vi "InsertIntoArray.vi"(0 "ROSCO Params":T3, 1 "ArrayPairs":T1={"iStatus"={"Index"=0, "Value"=0.0}, "TIME"={"Index"=1, "Value"=0.0}, "DT"={"Index"=2, "Value"=0.0}, "BL_PITCH"={"Index"=3, "Value"=0.0}, "VS_MECHGENPWR"={"Index"=13, "Value"=0.0}, "VS_GENPWR"={"Index"=14, "Value"=0.0}, "GEN_SPEED"={"Index"=19, "Value"=0.0}, "ROTOR_SPEED"={"Index"=20, "Value"=0.0}, "GENTQMEAS"={"Index"=22, "Value"=0.0}, "Y_M"={"Index"=23, "Value"=0.0}, "HORWINDV"={"Index"=26, "Value"=0.0}, "ROOTMOOP1"={"Index"=29, "Value"=0.0}, "ROOTMOOP2"={"Index"=30, "Value"=0.0}, "BL_PITCH2"={"Index"=32, "Value"=0.0}, "BL_PITCH3"={"Index"=33, "Value"=0.0}, "ROOTMOOP3"={"Index"=31, "Value"=0.0}, "AVCMSG_SIZE"={"Index"=48, "Value"=0.0}, "INFILE_SIZE "={"Index"=49, "Value"=0.0}, "OUTFILE_SIZE "={"Index"=50, "Value"=0.0}, "FA_ACC"={"Index"=52, "Value"=0.0}, "NUM_BLADES"={"Index"=60, "Value"=0.0}, "OUT_BL_PITCH"={"Index"=44, "Value"=0.0}, "OUT_TORQUE"={"Index"=46, "Value"=0.0}, "OUT_AERODYN_TQ"={"Index"=89, "Value"=0.0}}, 3 "error in (no error)":errorcluster, 4 "index":i32, 6 "number":sgl) -> (7 "ROSCO Params Out":T3, 8 "ArrayPairs Out":T1={"iStatus"={"Index"=0, "Value"=0.0}, "TIME"={"Index"=1, "Value"=0.0}, "DT"={"Index"=2, "Value"=0.0}, "BL_PITCH"={"Index"=3, "Value"=0.0}, "VS_MECHGENPWR"={"Index"=13, "Value"=0.0}, "VS_GENPWR"={"Index"=14, "Value"=0.0}, "GEN_SPEED"={"Index"=19, "Value"=0.0}, "ROTOR_SPEED"={"Index"=20, "Value"=0.0}, "GENTQMEAS"={"Index"=22, "Value"=0.0}, "Y_M"={"Index"=23, "Value"=0.0}, "HORWINDV"={"Index"=26, "Value"=0.0}, "ROOTMOOP1"={"Index"=29, "Value"=0.0}, "ROOTMOOP2"={"Index"=30, "Value"=0.0}, "BL_PITCH2"={"Index"=32, "Value"=0.0}, "BL_PITCH3"={"Index"=33, "Value"=0.0}, "ROOTMOOP3"={"Index"=31, "Value"=0.0}, "AVCMSG_SIZE"={"Index"=48, "Value"=0.0}, "INFILE_SIZE "={"Index"=49, "Value"=0.0}, "OUTFILE_SIZE "={"Index"=50, "Value"=0.0}, "FA_ACC"={"Index"=52, "Value"=0.0}, "NUM_BLADES"={"Index"=60, "Value"=0.0}, "OUT_BL_PITCH"={"Index"=44, "Value"=0.0}, "OUT_TORQUE"={"Index"=46, "Value"=0.0}, "OUT_AERODYN_TQ"={"Index"=89, "Value"=0.0}}, 10 "error out":errorcluster)   [LabVIEW 2018]
uses:
  Clusters/RoscoParams.ctl
  Clusters/ArrayPairs.ctl
  Clusters/SwapArrayCluster.ctl
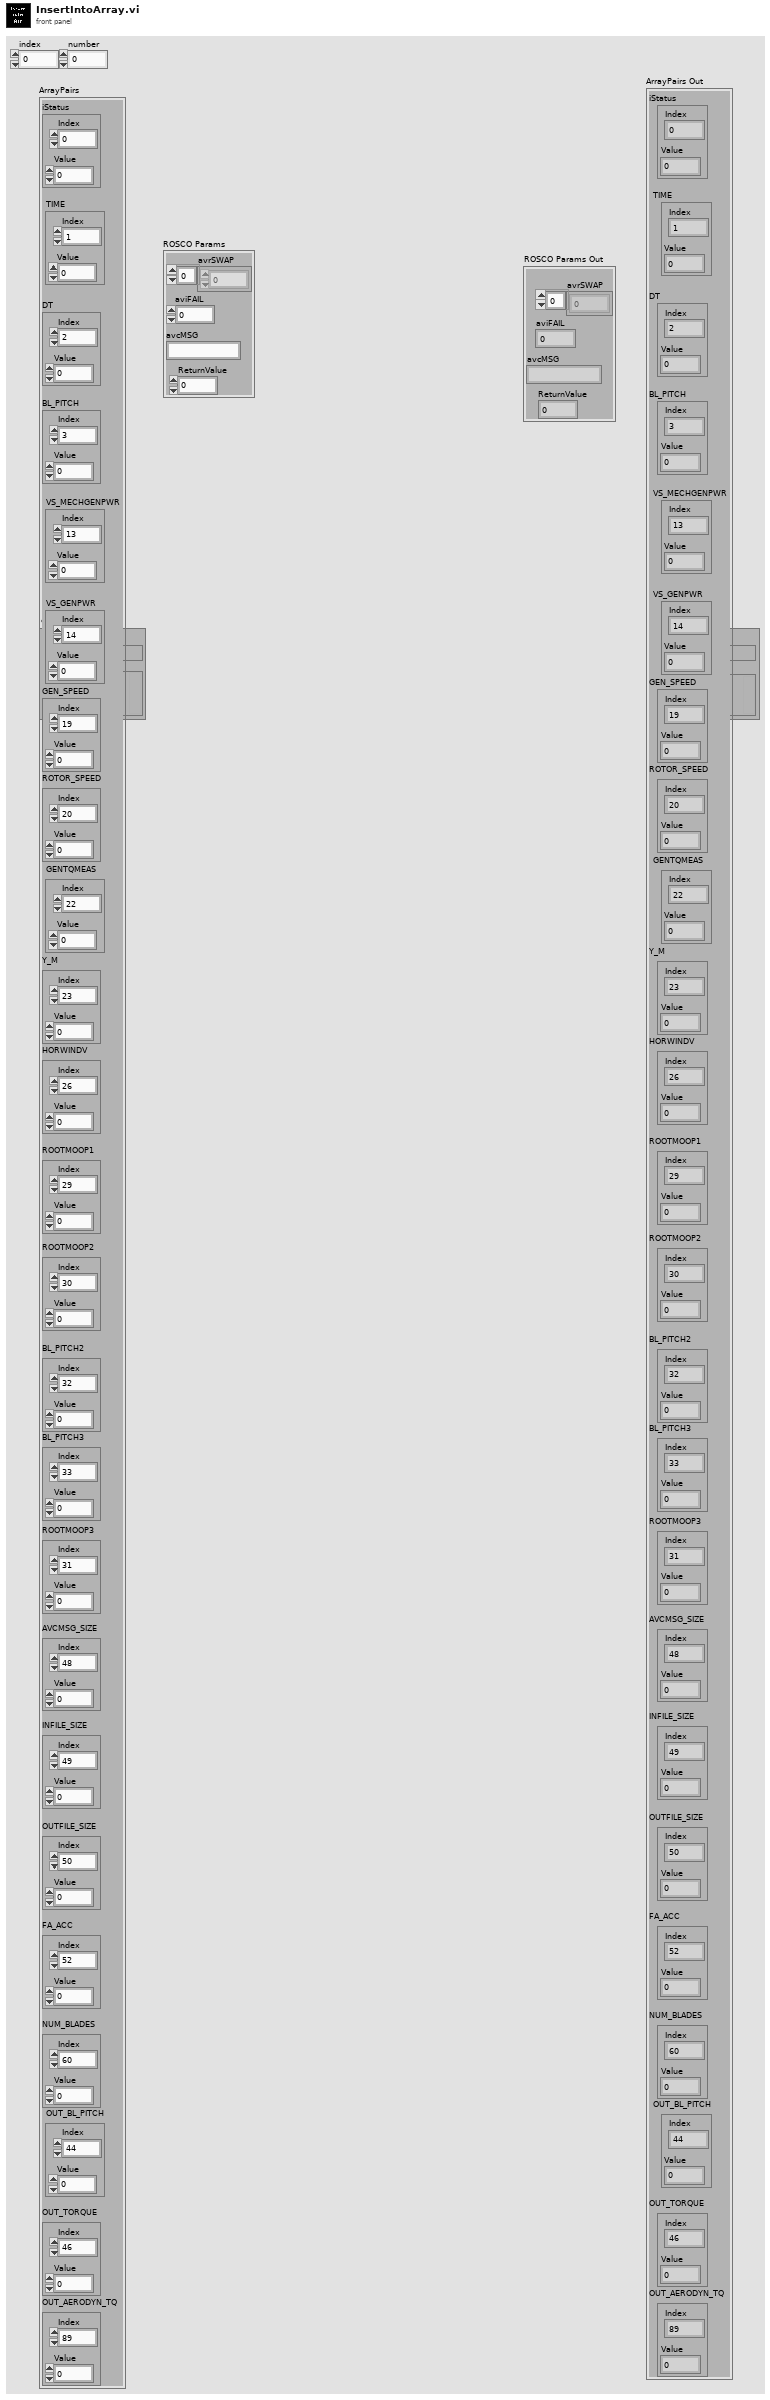
[diagram p1: front panel]
types:
  T1 = typedef "ArrayPairs.ctl" = cluster{"iStatus":T2, "TIME":T2, "DT":T2, "BL_PITCH":T2, "VS_MECHGENPWR":T2, "VS_GENPWR":T2, "GEN_SPEED":T2, "ROTOR_SPEED":T2, "GENTQMEAS":T2, "Y_M":T2, "HORWINDV":T2, "ROOTMOOP1":T2, "ROOTMOOP2":T2, "BL_PITCH2":T2, "BL_PITCH3":T2, "ROOTMOOP3":T2, "AVCMSG_SIZE":T2, "INFILE_SIZE ":T2, "OUTFILE_SIZE ":T2, "FA_ACC":T2, "NUM_BLADES":T2, "OUT_BL_PITCH":T2, "OUT_TORQUE":T2, "OUT_AERODYN_TQ":T2}
  T2 = typedef "SwapArrayCluster.ctl" = cluster{"Index":i32, "Value":sgl}
  T3 = typedef "RoscoParams.ctl" = cluster{"avrSWAP":sgl[], "aviFAIL":i32, "avcMSG":string, "ReturnValue":i32}
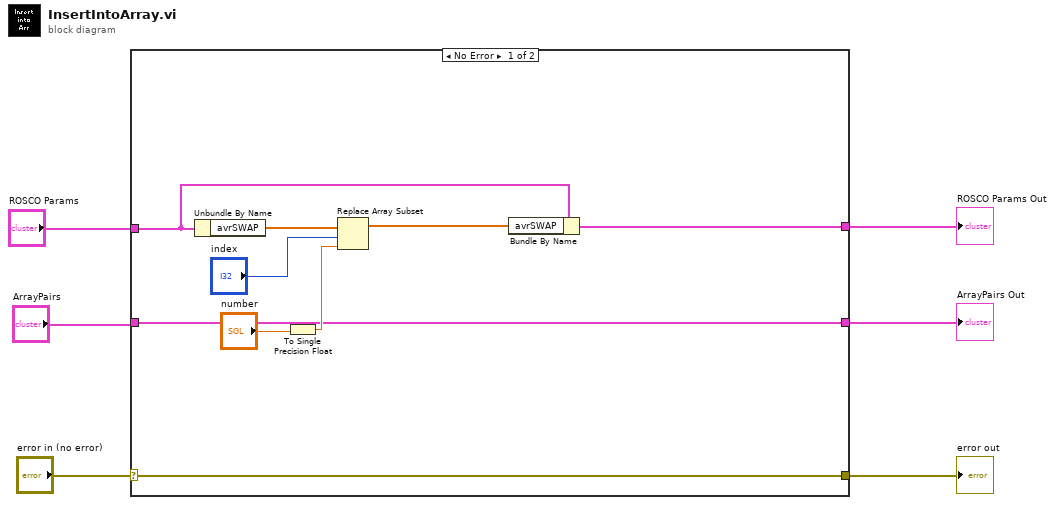
[diagram p0: block diagram]
diagram:
  n1 = case shown="No Error" "error in (no error)" {
    selector: "error in (no error)" -> [w15 w17]
    tunnel: "ROSCO Params" -> [w12 w18]
    tunnel: [w15 w17] -> w4
    tunnel: [w10 w18] -> w3
    tunnel: "ArrayPairs" -> [w9 w16]
    tunnel: [w9 w16] -> w1
    frame No Error {
      n2 = Unbundle By Name(w12) -> ("avrSWAP"=w14:sgl[])
      n3 = To Single Precision Float(number="number") -> (single precision float=w13:sgl)
      n4 = Replace Array Subset(array=w14, new element=w13, index="index") -> (w11:sgl[])
      n5 = Bundle By Name(cluster=w12, "avrSWAP"=w11) -> (w10:T3)
    }
    frame Error {
    }
  }
  "error out" <- w4
  "ROSCO Params Out" <- w3
  "ArrayPairs Out" <- w1
